vi "BoxBegin.vi"(8 "error in (no error)":errorcluster) -> (0 "error out":errorcluster)   [LabVIEW 2023]
uses:
  <vilib>/Rock Robotics/WPI/ThirdParty/REV Robotics/REVLib/Typedef/Spark MAX Idle Mode.ctl
  <vilib>/Rock Robotics/SystemInterfaces/DIO/FPGA_DIOChannel.ctl
  <vilib>/Rock Robotics/WPI/ThirdParty/REV Robotics/REVLib/SubVI/Public/SPARK Open Brushless.vi
  <vilib>/Rock Robotics/WPI/ThirdParty/REV Robotics/REVLib/SubVI/Public/SPARK Configure Basic Idle Mode.vi
  <vilib>/Rock Robotics/WPI/ThirdParty/REV Robotics/REVLib/SubVI/Public/SPARK Configure Basic Ramp Rate.vi
  <vilib>/Rock Robotics/WPI/ThirdParty/REV Robotics/REVLib/SubVI/Public/SPARK Configure Power Smart Current Limit.vi
  <vilib>/Rock Robotics/WPI/ThirdParty/REV Robotics/REVLib/SubVI/Public/SPARK Configure Encoder Conversion Factors.vi
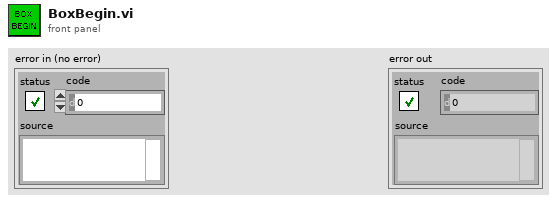
[diagram p1: front panel]
types:
  T1 = typedef "Spark MAX Idle Mode.ctl" = enum16{"Coast", "Brake"}
  T2 = typedef "FPGA_DIOChannel.ctl" = enum8{"DIO 0", "DIO 1", "DIO 2", "DIO 3", "DIO 4", "DIO 5", "DIO 6", "DIO 7", "DIO 8", "DIO 9", "DIO MXP 0", "DIO MXP 1", "DIO MXP 2", "DIO MXP 3", "DIO MXP 4", "DIO MXP 5", "DIO MXP 6", "DIO MXP 7", "DIO MXP 8", "DIO MXP 9", "DIO MXP 10", "DIO MXP 11", "DIO MXP 12", "DIO MXP 13", "DIO MXP 14", "DIO MXP 15", "SPI Port CS1", "SPI Port CS2", "SPI Port CS3", "SPI Port MISO", "SPI Port MOSI", "Invalid"}
  T3 = typedef "WPI_MotorControlDeviceRef.ctl" = cluster{"DeviceStatus":errorcluster, "Type":T4, "PWM":cluster{"PWM Channel":T5, "DeadBand":T6}, "CAN":cluster{"Device Number":u8, "SetOutput VI Ref":variant, "GetOutput VI Ref":variant, "Enable VI Ref":variant, "Disable VI Ref":variant, "Data":variant}, "Invert":bool, "DIO PWM":cluster{"PWM \"Enable\" Channel":T5, "DIOChannel":T2, "PWM Rate":dbl}}
  T4 = typedef "WPI_MotorControlType.ctl" = enum16{"PWM", "CAN", "DIO PWM"}
  T5 = typedef "FPGA_DIOPWMChannel.ctl" = enum8{"PWM 0", "PWM 1", "PWM 2", "PWM 3", "PWM 4", "PWM 5", "PWM 6", "PWM 7", "PWM 8", "PWM 9", "PWM MXP 0", "PWM MXP 1", "PWM MXP 2", "PWM MXP 3", "PWM MXP 4", "PWM MXP 5", "PWM MXP 6", "PWM MXP 7", "PWM MXP 8", "PWM MXP 9", "Invalid"}
  T6 = typedef "WPI_PWMDeadband.ctl" = cluster{"Name":string, "maxPositivePwm":i32, "minPositivePwm":i32, "centerPwm":i32, "maxNegativePwm":i32, "minNegativePwm":i32, "angularRange":u16}
  T7 = typedef "WPI_DigitalInputDevRef.ctl" = cluster{"DevStatus":errorcluster, "DIO Channel":T2}
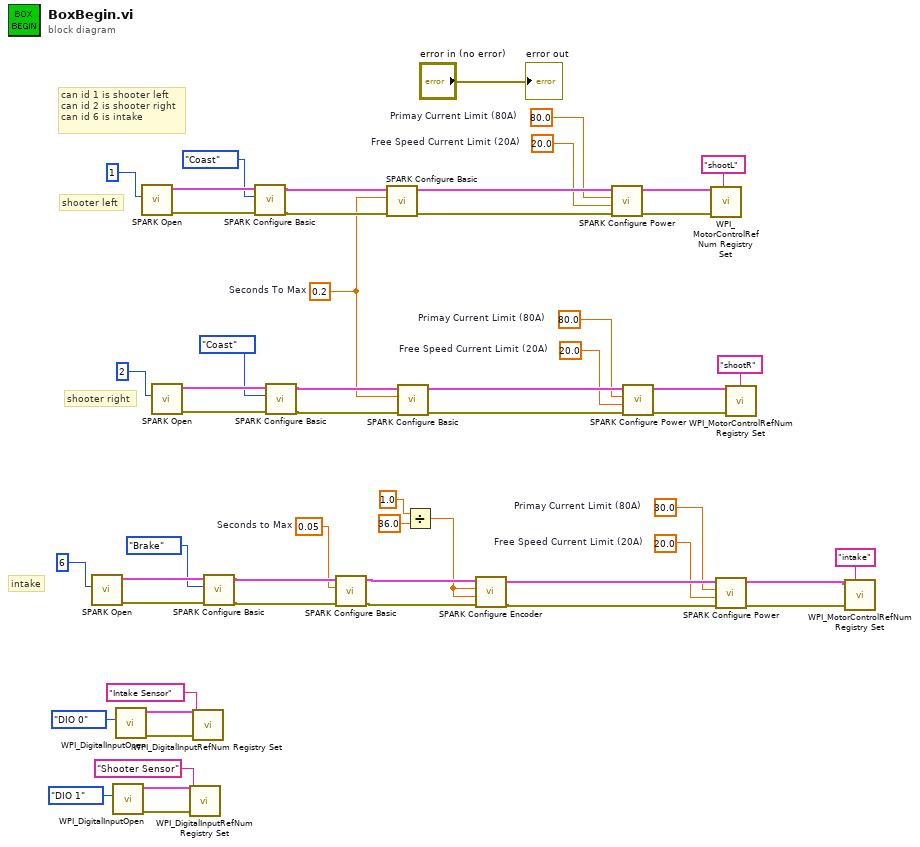
[diagram p0: block diagram]
diagram:
  w30 = 20.0  # Free Speed Current Limit (20A)
  w31 = 80.0  # Primay Current Limit (80A)
  w18 = 20.0  # Free Speed Current Limit (20A)
  w19 = 80.0  # Primay Current Limit (80A)
  w1 = 20.0  # Free Speed Current Limit (20A)
  w2 = 30.0  # Primay Current Limit (80A)
  w11 = 0.05  # Seconds to Max
  w20 = 0.2  # Seconds To Max
  # "intake"
  # "shooter right"
  # "shooter left"
  # "can id 1 is shooter left\ncan id 2 is shooter right\ncan id 6 is intake"
  n1 = call-poly <vilib>:"SPARK Open.vi"("Device Number"=6) -> ("error out"=w12:errorcluster, "MotorControlDeviceRef"=w13:T3)  [unwired: 9 in]
  n2 = call <vilib>:"WPI_DigitalInputOpen.vi"("DIO Channel"=FPGA_DIOChannel."DIO 1") -> ("error out"=w42:errorcluster, "DigitalInputDevRef"=w41:T7)  [unwired: 9 in]
  n3 = call <vilib>:"WPI_DigitalInputOpen.vi"("DIO Channel"=FPGA_DIOChannel."DIO 0") -> ("error out"=w46:errorcluster, "DigitalInputDevRef"=w45:T7)  [unwired: 9 in]
  n4 = call-poly <vilib>:"SPARK Open.vi"("Device Number"=1) -> ("error out"=w37:errorcluster, "MotorControlDeviceRef"=w38:T3)  [unwired: 9 in]
  n5 = call-poly <vilib>:"SPARK Open.vi"("Device Number"=2) -> ("error out"=w22:errorcluster, "MotorControlDeviceRef"=w23:T3)  [unwired: 9 in]
  n6 = call <vilib>:"WPI_DigitalInputRefNum Registry Set.vi"("error in (no error)"=w42, "refnum name"="Shooter Sensor", "DigitalInputDevRef"=w41) -> ()  [unwired: 7 in, 2 out]
  n7 = call <vilib>:"WPI_DigitalInputRefNum Registry Set.vi"("error in (no error)"=w46, "refnum name"="Intake Sensor", "DigitalInputDevRef"=w45) -> ()  [unwired: 7 in, 2 out]
  n8 = call-poly <vilib>:"SPARK Configure Basic.vi"("error in (no error)"=w12, "Idle Mode"=Spark_MAX_Idle_Mode."Brake", "MotorControlDeviceRef in"=w13) -> ("error out"=w14:errorcluster, "MotorControlDeviceRef out"=w15:T3)  [unwired: 7 in]
  n9 = call-poly <vilib>:"SPARK Configure Basic.vi"("error in (no error)"=w37, "Idle Mode"=Spark_MAX_Idle_Mode."Coast", "MotorControlDeviceRef in"=w38) -> ("error out"=w34:errorcluster, "MotorControlDeviceRef out"=w35:T3)  [unwired: 7 in]
  n10 = call-poly <vilib>:"SPARK Configure Basic.vi"("error in (no error)"=w22, "Idle Mode"=Spark_MAX_Idle_Mode."Coast", "MotorControlDeviceRef in"=w23) -> ("error out"=w26:errorcluster, "MotorControlDeviceRef out"=w27:T3)  [unwired: 7 in]
  n11 = call-poly <vilib>:"SPARK Configure Basic.vi"("error in (no error)"=w14, "Seconds from neutral to full (0)"=w11, "MotorControlDeviceRef in"=w15) -> ("error out"=w8:errorcluster, "MotorControlDeviceRef"=w9:T3)  [unwired: 7 in]
  n12 = call-poly <vilib>:"SPARK Configure Basic.vi"("error in (no error)"=w34, "Seconds from neutral to full (0)"=w20, "MotorControlDeviceRef in"=w35) -> ("error out"=w32:errorcluster, "MotorControlDeviceRef"=w33:T3)  [unwired: 7 in]
  n13 = call-poly <vilib>:"SPARK Configure Basic.vi"("error in (no error)"=w26, "Seconds from neutral to full (0)"=w20, "MotorControlDeviceRef in"=w27) -> ("error out"=w24:errorcluster, "MotorControlDeviceRef"=w25:T3)  [unwired: 7 in]
  n14 = Divide(x=1.0, y=36.0) -> (x/y=w7:dbl)
  n15 = call-poly <vilib>:"SPARK Configure Encoder.vi"("error in"=w8, "Velocity Conversion Factor"=w7, "Position Conversion Factor"=w7, "MotorControlDeviceRef in"=w9) -> ("error out"=w5:errorcluster, "MotorControlDeviceRef out"=w6:T3)  [unwired: 6 in]
  n16 = call-poly <vilib>:"SPARK Configure Power.vi"("error in (no error)"=w32, "Free Speed Current Limit (20A)"=w30, "Primay Current Limit (80A)"=w31, "MotorControlDeviceRef in"=w33) -> ("error out"=w28:errorcluster, "MotorControlDeviceRef out"=w29:T3)  [unwired: 6 in]
  n17 = call-poly <vilib>:"SPARK Configure Power.vi"("error in (no error)"=w24, "Free Speed Current Limit (20A)"=w18, "Primay Current Limit (80A)"=w19, "MotorControlDeviceRef in"=w25) -> ("error out"=w16:errorcluster, "MotorControlDeviceRef out"=w17:T3)  [unwired: 6 in]
  n18 = call <vilib>:"WPI_MotorControlRefNum Registry Set.vi"("error in (no error)"=w28, "refnum name"="shootL", "MotorControlDevRef"=w29) -> ()  [unwired: 7 in, 2 out]
  n19 = call-poly <vilib>:"SPARK Configure Power.vi"("error in (no error)"=w5, "Free Speed Current Limit (20A)"=w1, "Primay Current Limit (80A)"=w2, "MotorControlDeviceRef in"=w6) -> ("error out"=w3:errorcluster, "MotorControlDeviceRef out"=w4:T3)  [unwired: 6 in]
  n20 = call <vilib>:"WPI_MotorControlRefNum Registry Set.vi"("error in (no error)"=w16, "refnum name"="shootR", "MotorControlDevRef"=w17) -> ()  [unwired: 7 in, 2 out]
  n21 = call <vilib>:"WPI_MotorControlRefNum Registry Set.vi"("error in (no error)"=w3, "refnum name"="intake", "MotorControlDevRef"=w4) -> ()  [unwired: 7 in, 2 out]
  "error out" <- "error in (no error)"
